vi "anglewithatan2.vi"(9 "mic3":dbl, 10 "mic2":dbl, 11 "mic1":dbl) -> (3 "angle":dbl)   [LabVIEW 2014]
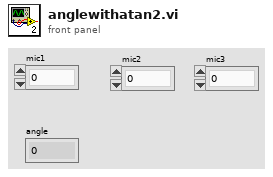
[diagram p1: front panel]
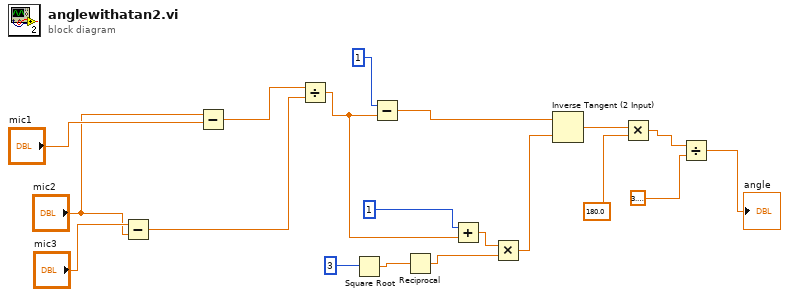
[diagram p0: block diagram]
diagram:
  n1 = Subtract(x="mic3", y="mic2") -> (x-y=w13:dbl)
  n2 = Subtract(x="mic2", y="mic1") -> (x-y=w14:dbl)
  n3 = Divide(x=w14, y=w13) -> (x/y=w9:dbl)
  n4 = Square Root(x=3) -> (sqrt(x)=w18:dbl)
  n5 = Subtract(x=1, y=w9) -> (x-y=w11:dbl)
  n6 = Reciprocal(x=w18) -> (1/x=w8:dbl)
  n7 = Add(x=1, y=w9) -> (x+y=w7:dbl)
  n8 = Multiply(x=w7, y=w8) -> (x*y=w6:dbl)
  n9 = Inverse Tangent (2 Input)(1:w6, 2:w11) -> (0:w1:dbl)
  n10 = Multiply(x=w1, y=180.0) -> (x*y=w4:dbl)
  n11 = Divide(x=w4, y=3.141592653589793) -> (x/y=→"angle":dbl)
